vi "Set Class Control Label.vi"(8 "error in (no error)":errorcluster, 10 "Class Name":string, 11 "vi reference in":refnum<vi>) -> (0 "error out":errorcluster, 3 "vi reference out":refnum<vi>)   [LabVIEW 2020, in "Message Maker.lvlib"]
uses:
  Message Maker.lvlib
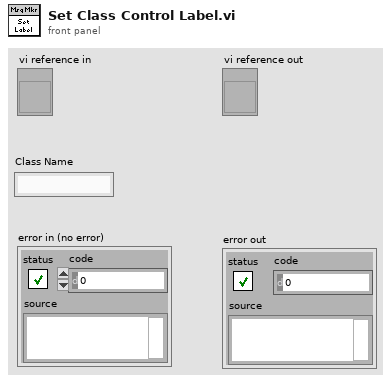
[diagram p1: front panel]
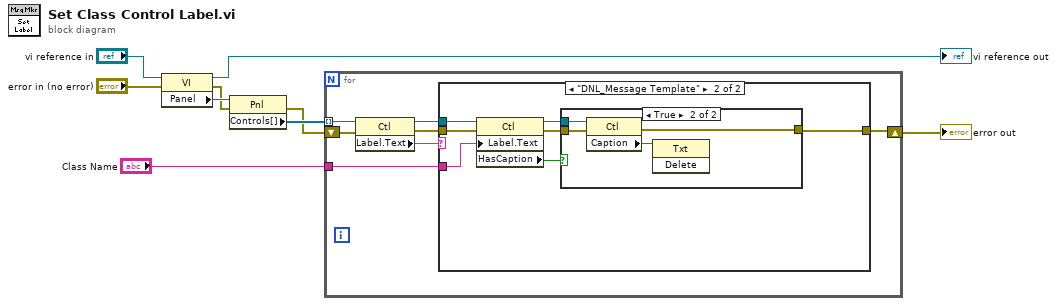
[diagram p0: block diagram]
diagram:
  n1 = property class="VI"(reference="vi reference in", error in="error in (no error)") -> (reference out=→"vi reference out":refnum<vi>, error out=w6:errorcluster, "Panel"=w8:refnum<vi>)
  n2 = property class="Pnl"(reference=w8, error in=w6) -> (error out=w5:errorcluster, "Controls[]"=w7:refnum<vi>[])  [unwired: 1 out]
  n3 = for {
    tunnel: w7 -> [w16] mode=indexing
    shift-right: [w11] -> w1
    shift-left: w5 -> [w13]
    tunnel: "Class Name" -> [w10]
    n4 = property class="Ctl"(reference=w16, error in=w13) -> (reference out=w14:refnum<vi>, error out=w12:errorcluster, "Label.Text"=w15:string)
    n5 = case shown="\"DNL_Message Template\"" w15 {
      tunnel: w14 -> [_ w19]
      tunnel: w12 -> [w17 w21]
      tunnel: [w17 w20] -> w11
      tunnel: w10 -> [_ w18]
      frame Default {
      }
      frame "DNL_Message Template" {
        n6 = property class="Ctl"(reference=w19, error in=w21, "Label.Text"=w18) -> (reference out=w22:refnum<vi>, error out=w23:errorcluster, "HasCaption"=w24:bool)
        n7 = case shown="True" w24 {
          tunnel: w22 -> [_ w28]
          tunnel: w23 -> [w25 w27]
          tunnel: [w25 w26] -> w20
          frame False {
          }
          frame True {
            n8 = property class="Ctl"(reference=w28, error in=w27) -> (error out=w26:errorcluster, "Caption"=w29:refnum<vi>)  [unwired: 1 out]
            n9 = invoke class="Txt" method="Delete"(reference=w29) -> ()  [unwired: 2 in, 3 out]
          }
        }
      }
    }
  }
  "error out" <- w1
